vi "Explain.vi"(8 "error in (no error)":errorcluster, 10 "Verbose Explanation":string, 11 "Assert in":refnum<class "Assert.lvclass">) -> (0 "error out":errorcluster, 3 "Assert out":refnum<class "Assert.lvclass">)   [LabVIEW 2013, in "Caraya.lvlib" / "Assert.lvclass"]
uses:
  Assert.lvclass
  Assert.lvclass/Assert.ctl
  Basic Test Manager/Basic Test Manager.lvclass
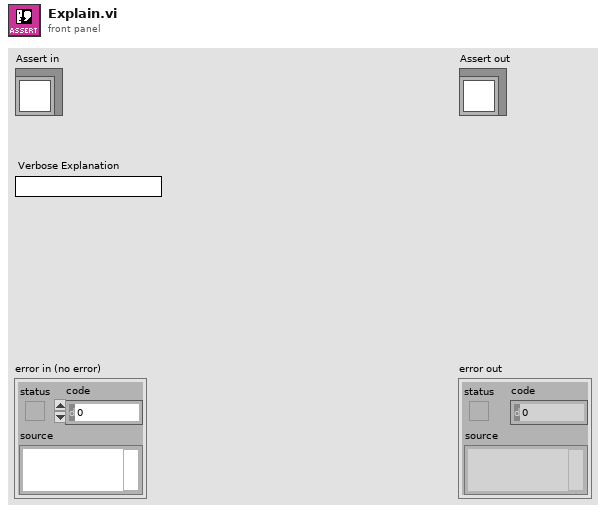
[diagram p1: front panel]
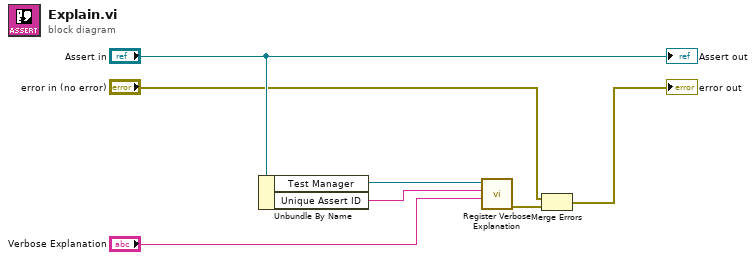
[diagram p0: block diagram]
diagram:
  n1 = Unbundle By Name("Assert in") -> ("Test Manager"=w7:refnum<class "Basic Test Manager.lvclass">, "Unique Assert ID"=w6:string)
  n2 = call-dynamic "Register Verbose Explanation.vi"("Explanation"="Verbose Explanation", "Unique ID"=w6, "Basic Test Manager in"=w7) -> ("error out"=w5:errorcluster)  [unwired: 7 in, 1 out]
  n3 = Merge Errors("error in (no error)", w5) -> (→"error out":errorcluster)
  "Assert out" <- "Assert in"
